vi "Read MUS Data.vi"(11 "Sound LUMP IN":u8[](array[numeric])) -> (0 "instr list":u8[](array[numeric]), 1 "CHAN_total":u16, 2 "Identifier":string, 3 "MUS_Data_out":u8[](array[numeric]))   [LabVIEW 2014]
panel:
  out "number of instr":u16
  out "2nd channels":u16
  out "1st channels":u16
  out "header len":u16
  out "music len":u16
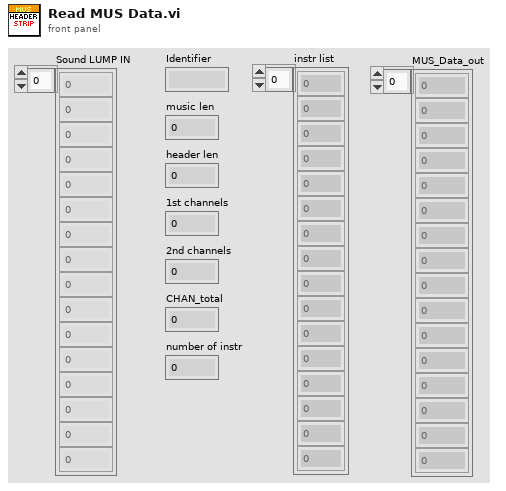
[diagram p1: front panel]
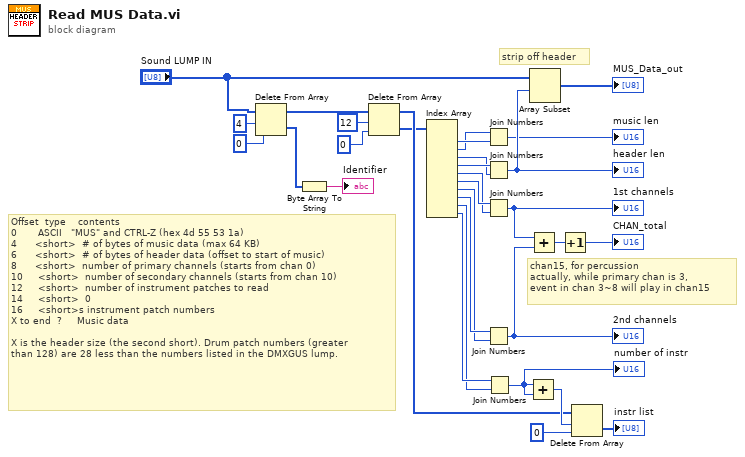
[diagram p0: block diagram]
diagram:
  # "chan15, for percussion\nactually, while primary chan is 3,\nevent in chan 3~8 will play in chan15"
  # "strip off header"
  # "Offset  type    contents\n0       ASCII   \"MUS\" and CTRL-Z (hex 4d 55 53 1a)\n4      <short>  # of bytes of music data (max 64 KB)\n6      <short>  # of bytes of header data (offset to start of music)\n8      <short>  number of primary channels (starts from chan 0)\n10     <short>  number of secondary channels (starts from chan 10)\n12     <short>  number of instrument patches to read\n14     <short>  0\n16     <short>s instrument patch numbers\nX to end  ?     Music data\n\nX is the header size (the second short). Drum patch numbers (greater\nthan 128) are 28 less than the numbers listed in the DMXGUS lump."
  n1 = Delete From Array(array="Sound LUMP IN", length=4, index=0) -> (deleted portion=w2:u8[], array with subset deleted=w25:u8[])
  n2 = Byte Array To String(unsigned byte array=w2) -> (string=→"Identifier":string)
  n3 = Delete From Array(array=w25, length=12, index=0) -> (deleted portion=w11:u8[], array with subset deleted=w23:u8[])
  n4 = Index Array(array=w11) -> (element #1=w13:u8, element #2=w12:u8, element #3=w14:u8, element #4=w15:u8, element #5=w16:u8, element #6=w17:u8, element #7=w18:u8, element #8=w19:u8, element #9=w20:u8, element #10=w21:u8)  [unwired: 10 in]
  n5 = Join Numbers(hi=w12, lo=w13) -> ((hi.lo)=→"music len":u16)
  n6 = Join Numbers(hi=w15, lo=w14) -> ((hi.lo)=w24:u16)
  "header len" <- w24
  n7 = Join Numbers(hi=w17, lo=w16) -> ((hi.lo)=w29:u16)
  "1st channels" <- w29
  n8 = Join Numbers(hi=w19, lo=w18) -> ((hi.lo)=w28:u16)
  "2nd channels" <- w28
  n9 = Join Numbers(hi=w21, lo=w20) -> ((hi.lo)=w30:u16)
  "number of instr" <- w30
  n10 = Add(x=w30, y=w30) -> (x+y=w31:u16)
  n11 = Add(x=w29, y=w28) -> (x+y=w27:u16)
  n12 = Array Subset(array="Sound LUMP IN", index=w24) -> (→"MUS_Data_out":u8[])  [unwired: 1 in]
  n13 = Increment(x=w27) -> (x+1=→"CHAN_total":u16)
  n14 = Delete From Array(array=w23, length=w31, index=0) -> (deleted portion=→"instr list":u8[])  [unwired: 1 out]
